vi "Pre Launch Init.vi"(11 "Actor Nest in":refnum<class "Actor Nest.lvclass">) -> (0 "error out":errorcluster, 3 "Actor Nest out":refnum<class "Actor Nest.lvclass">)   [LabVIEW 2012, in "Actor Nest.lvlib" / "Actor Nest.lvclass"]
doc: "(<B>Filename</B>: Actor Framework.lvlib:Actor.lvclass:Pre Launch Init.vi)\n\nDefines behavior that occurs after the Launch Actor method is invoked but before the actor's Actor Core method begins running.\n\nThe Pre Launch Init method is guaranteed to finish before the Launch Actor method returns to its caller and before the actor itself receives any messages. Any references that the Pre Launch Init method obtains are guaranteed to have the same lifetime as the actor itself. Any errors that the Pre Launch Init method returns will abort the launch.\n\nBy default, this method does nothing. A descendant class may override it to define behavior."
uses:
  Actor Nest.lvclass
  Actor Nest.lvclass/Actor Nest.ctl
  <vilib>/ActorFramework/Actor/Actor.lvclass
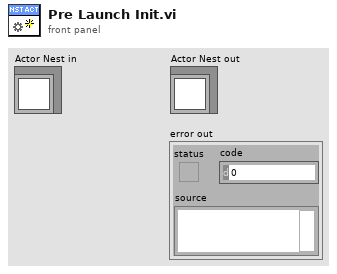
[diagram p1: front panel]
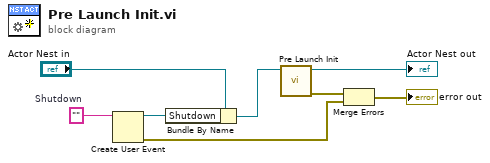
[diagram p0: block diagram]
diagram:
  w7 = ""  # Shutdown
  n1 = Create User Event(user event datatype=w7) -> (user event=w6:refnum<user-event>, error out=w2:errorcluster)  [unwired: 1 in]
  n2 = Bundle By Name(cluster="Actor Nest in", "Shutdown"=w6) -> (w4:refnum<class "Actor Nest.lvclass">)
  n3 = call-parent "Pre Launch Init.vi"("Actor in"=w4) -> ("error out"=w3:errorcluster, "Actor out"=→"Actor Nest out":refnum<class "Actor Nest.lvclass">)  [unwired: 9 in]
  n4 = Merge Errors(w3, w2) -> (→"error out":errorcluster)
